vi "API String - Float Format String.vi"(8 "Error in":errorcluster caption="Error in (no error)") -> (0 "Error out":errorcluster, 3 "Float Format String":string)   [LabVIEW 2017, in "API String Arguments Support.lvlib"]
uses:
  API String Arguments Support.lvlib
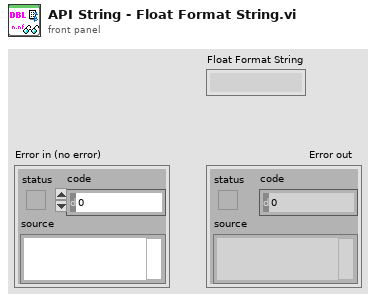
[diagram p1: front panel]
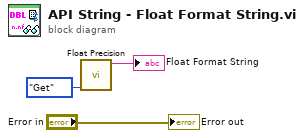
[diagram p0: block diagram]
diagram:
  n1 = call "Float Precision.vi"("Enum"=enum16{"Set", "Get"}."Get") -> ("Format String"=→"Float Format String":string)  [unwired: 10 in]
  "Error out" <- "Error in"
